vi "Get CAN Configuration.vi"(8 "error in (no error)":errorcluster, 11 "Ethernet in":refnum<class "ENET_BS1200.lvclass">) -> (0 "error out":errorcluster, 1 "Configuration Error?":bool, 2 "CAN Settings":T1, 3 "Ethernet out":refnum<class "ENET_BS1200.lvclass">)   [LabVIEW 2021, in "BS120x Driver.lvlib" / "ENET_BS1200.lvclass"]
doc: "Retrieve Battery Simulator 1200 CAN settings.\n(c) 2019 Bloomy Controls, Inc. All rights reserved."
uses:
  ENET_BS1200.lvclass
  TypeDefs/CAN Settings.ctl
  <vilib>/WebDAVClient/Advanced/Get Buffer.vi
  ENET_BS1200.lvclass/ENET_BS1200.ctl
  <vilib>/WebDAVClient/NI_WebDAV.lvlib
  BS120x.lvclass
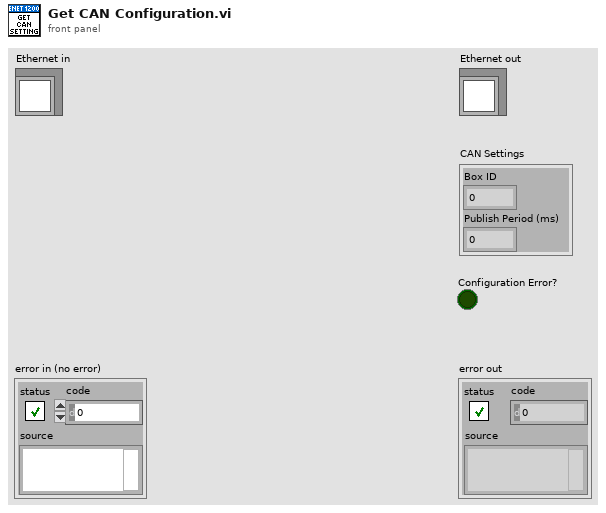
[diagram p1: front panel]
types:
  T1 = typedef "BS120x Driver.lvlib/BS120x.lvclass/CAN Settings.ctl" = cluster{"Box ID":i32, "Publish Period (ms)":i32}
  T2 = typedef "NI_WebDAV.lvlib/SessionHandle.ctl" = refnum<k1>
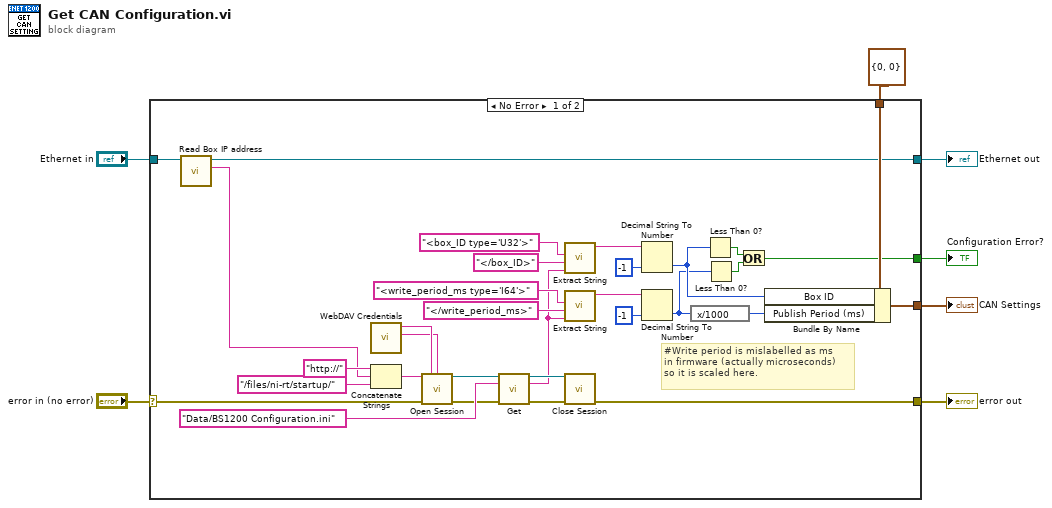
[diagram p0: block diagram]
diagram:
  n1 = case shown="No Error" "error in (no error)" {
    selector: "error in (no error)" -> [w35 w42]
    tunnel: [w30 w42] -> w6
    tunnel: [w9 w41] -> w4
    tunnel: "Ethernet in" -> [w10 w41]
    tunnel: [w38 w40] -> w2
    tunnel: T1 {"Box ID"=0, "Publish Period (ms)"=0} ("CAN Settings") -> [w39 w40]
    tunnel: [w12 _] -> w1
    frame No Error {
      # "#Write period is mislabelled as ms\nin firmware (actually microseconds)\nso it is scaled here."
      n2 = call-dynamic "Read Box IP address.vi"("ENET_BS120x in"=w10) -> ("Box IP address"=w8:string, "ENET_BS120x out"=w9:refnum<class "ENET_BS1200.lvclass">)  [unwired: 8 in, 1 out]
      n3 = call "WebDAV Credentials.vi"() -> ("Password"=w33:string, "Username"=w34:string)  [unwired: 10 in]
      n4 = Concatenate Strings("http://" ("string"), w8, "/files/ni-rt/startup/" ("string")) -> (w32:string)
      n5 = call <vilib>:"Open Session.vi"("host uri prefix"=w32, "username"=w34, "password"=w33, "error in (no error)"=w35) -> ("session handle out"=w29:T2, "error out"=w28:errorcluster)  [unwired: 10 in]
      n6 = call-poly <vilib>:"Get.vi"("session handle"=w29, "relative uri"="Data/BS1200 Configuration.ini" ("string"), "error in (no error)"=w28) -> ("session handle out"=w27:T2, "data"=w11:string, "error out"=w24:errorcluster)  [unwired: 10 in]
      n7 = call "Extract String.vi"("Input String"=w11, "Text After String"="</box_ID>" ("regular expression"), "Text Before String"="<box_ID type='U32'>" ("regular expression")) -> ("Value String"=w19:string)  [unwired: 8 in]
      n8 = call "Extract String.vi"("Input String"=w11, "Text After String"="</write_period_ms>" ("regular expression"), "Text Before String"="<write_period_ms type='I64'>" ("regular expression")) -> ("Value String"=w21:string)  [unwired: 8 in]
      n9 = call <vilib>:"Close Session.vi"("session handle"=w27, "error in (no error)"=w24) -> ("error out"=w30:errorcluster)  [unwired: 13 in]
      n10 = Decimal String To Number(string=w19, default (0L)=-1 ("default (0 I32)")) -> (number=w16:i32)  [unwired: 1 in, 1 out]
      n11 = Decimal String To Number(string=w21, default (0L)=-1 ("default (0 I32)")) -> (number=w15:i32)  [unwired: 1 in, 1 out]
      n12 = expression code="x/1000"(w15) -> (w20:i32)
      n13 = Less Than 0?(x=w16) -> (x < 0?=w14:bool)
      n14 = Less Than 0?(x=w15) -> (x < 0?=w13:bool)
      n15 = Or(x=w14, y=w13) -> (x .or. y?=w12:bool)
      n16 = Bundle By Name(cluster=w39, "Box ID"=w16, "Publish Period (ms)"=w20) -> (w38:T1)
    }
    frame Error {
    }
  }
  "error out" <- w6
  "Ethernet out" <- w4
  "CAN Settings" <- w2
  "Configuration Error?" <- w1
